vi "grafica.vi"(0 "CabinaA":dbl, 1 "CabinaB":dbl) -> (2 "Graficas":cluster{"CabinaA":dbl, "CabinaB":dbl}(graph))   [LabVIEW 2021]
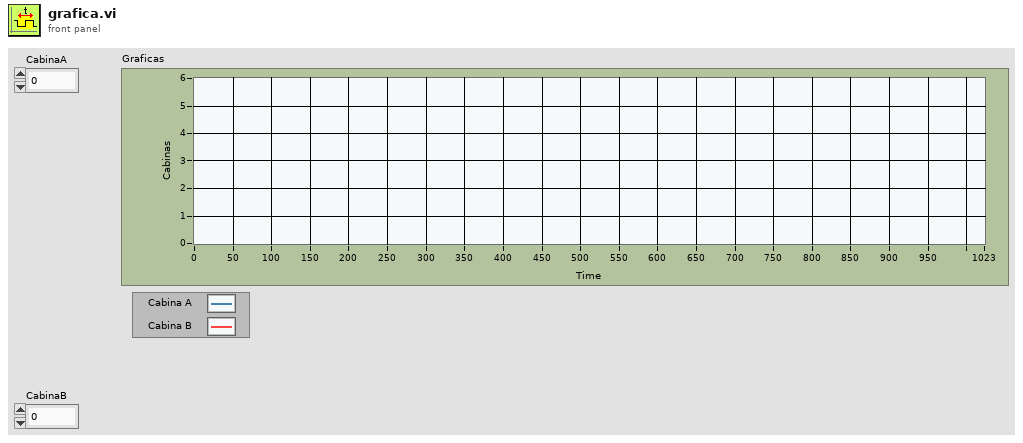
[diagram p1: front panel]
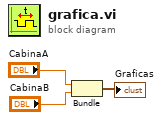
[diagram p0: block diagram]
diagram:
  n1 = Bundle("CabinaA"="CabinaA", "CabinaB"="CabinaB") -> (→"Graficas":cluster{"CabinaA":dbl, "CabinaB":dbl})  [unwired: 1 in]
